vi "SanityChecker.vi"(4 "MaxCone":dbl=58.0, 5 "Theta":dbl, 6 "Minimum dP":dbl=0.2, 7 "U":dbl, 9 "ZeroedPressures":dbl[](array[numeric]), 11 "ReductionError":i32) -> (1 "ErrorArray":bool[](array[boolean]), 2 "Plug in titles":string[](array[string])=["Good", "AllNegative", "dPTooSmall", "P1smallest", "FailedToReduce", "ExceedMaxCone", "U.LT.0"], 3 "CleanPoint":bool)   [LabVIEW 2013]
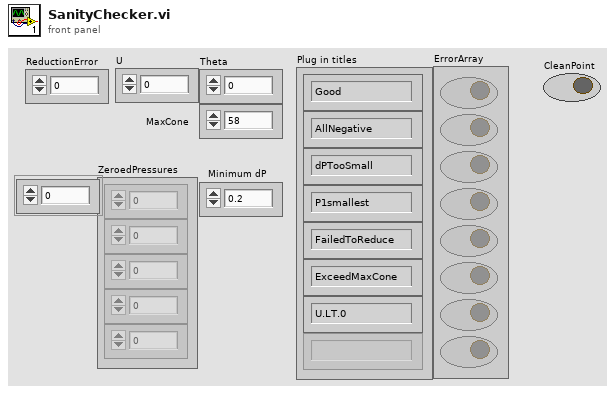
[diagram p1: front panel]
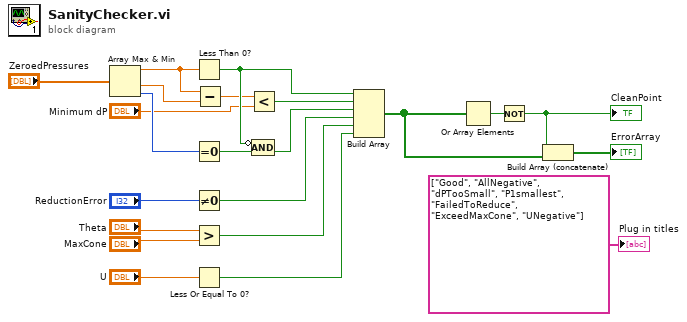
[diagram p0: block diagram]
diagram:
  n1 = Array Max & Min(array="ZeroedPressures") -> (max value=w5:dbl, min value=w6:dbl, min index (indices)=w17:i32)  [unwired: 1 out]
  n2 = Less Than 0?(x=w5) -> (x < 0?=w20:bool)
  n3 = Equal To 0?(x=w17) -> (x = 0?=w18:bool)
  n4 = Not Equal To 0?(x="ReductionError") -> (x != 0?=w13:bool)
  n5 = Greater?(x="Theta", y="MaxCone") -> (0:w14:bool)
  n6 = Less Or Equal To 0?(x="U") -> (x <= 0?=w22:bool)
  n7 = Subtract(x=w5, y=w6) -> (x-y=w7:dbl)
  n8 = Less?(x=w7, y="Minimum dP") -> (x < y?=w12:bool)
  n9 = Compound Arithmetic op=AND(invert w20, w18) -> (w19:bool)
  n10 = Build Array(w20, w12, w19, w13, w14, w22) -> (w16:bool[])
  n11 = Or Array Elements(Boolean array=w16) -> (logical OR=w15:bool)
  n12 = Not(x=w15) -> (.not. x?=w1:bool)
  "CleanPoint" <- w1
  n13 = Build Array (concatenate)(w1, w16) -> (→"ErrorArray":bool[])
  "Plug in titles" <- string[] ["Good", "AllNegative", "dPTooSmall", "P1smallest", "FailedToReduce", "ExceedMaxCone", "UNegative"] ("Plug in titles")
